vi "wave 3.vi"() -> ()   [LabVIEW 2011]
panel:
  out "XY Graph":cluster{dbl[], dbl[]}[](graph)
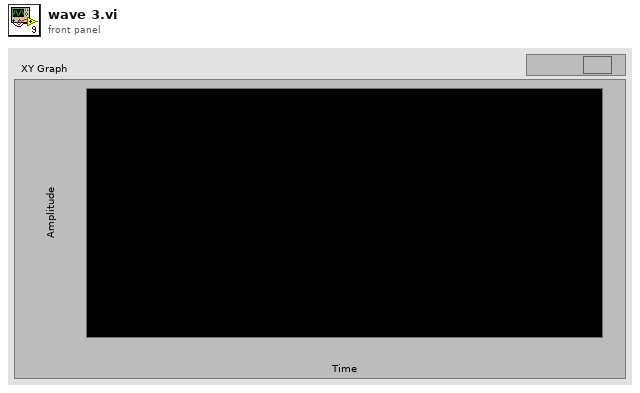
[diagram p1: front panel]
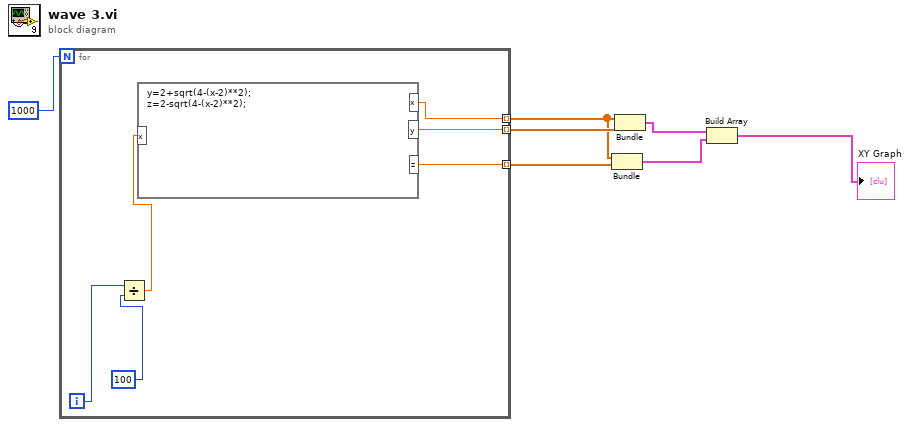
[diagram p0: block diagram]
diagram:
  n1 = for {
    N: 1000 -> [_]
    tunnel: [w12] -> w4 mode=indexing
    tunnel: [w11] -> w6 mode=indexing
    tunnel: [w10] -> w5 mode=indexing
    i -> [w9]
    n2 = Divide(x=w9, y=100) -> (x/y=w13:dbl)
    n3 = formula code="y=2+sqrt(4-(x-2)**2);\nz=2-sqrt(4-(x-2)**2);"("x"=w13) -> ("y"=w11:dbl, "z"=w10:dbl, "x"=w12:dbl)
  }
  n4 = Bundle(w4, w5) -> (w1:cluster{dbl[], dbl[]})  [unwired: 1 in]
  n5 = Bundle(w4, w6) -> (w2:cluster{dbl[], dbl[]})  [unwired: 1 in]
  n6 = Build Array(w2, w1) -> (→"XY Graph":cluster{dbl[], dbl[]}[])
